vi "Prepare Data for LSL.vi"(10 "Data Cluster":T1={"Status"="", "LSL Streaming"=FALSE, "channel_format"=1, "outlet"=0, "streaminfo"=0, "xml_ptr"=0, "LSL Listeners"=0, "LSL Listeners Query Counter"=0, "Data Chunk "={"counter"=0, "Data"=[]}, "Ch En Map"=[]} {"channel_format" items=["cft_float32"=1, "cft_double64"=2, "cft_string"=3, "cft_int32"=4, "cft_int16"=5, "cft_int8"=6, "cft_int64"=7, "cft_undefined"=0]}, 11 "WiBCI16T Data":T6 {"Reg Map"."ADS2" format="%x"; "Reg Map"."ADS1" format="%x"}) -> (2 "Data Chunk Size":i32, 3 "Prepared Data Array":dbl[][](array[numeric]))   [LabVIEW 2016, in "Lab Streaming Layer.lvlib"]
uses:
  Lab Streaming Layer.lvlib
  Acquisition/WiBCI16T_Data.ctl
  Acquisition/WiBCI16T_Status.ctl
  Acquisition/Reg_Map.ctl
  Module Data--cluster.ctl
  Custom Controls/lsl_channel_format.ctl
  Custom Controls/lsl_outlet.ctl
  Custom Controls/lsl_streaminfo.ctl
  Custom Controls/lsl_xml_ptr.ctl
  Acquisition/Acquisition.lvlib
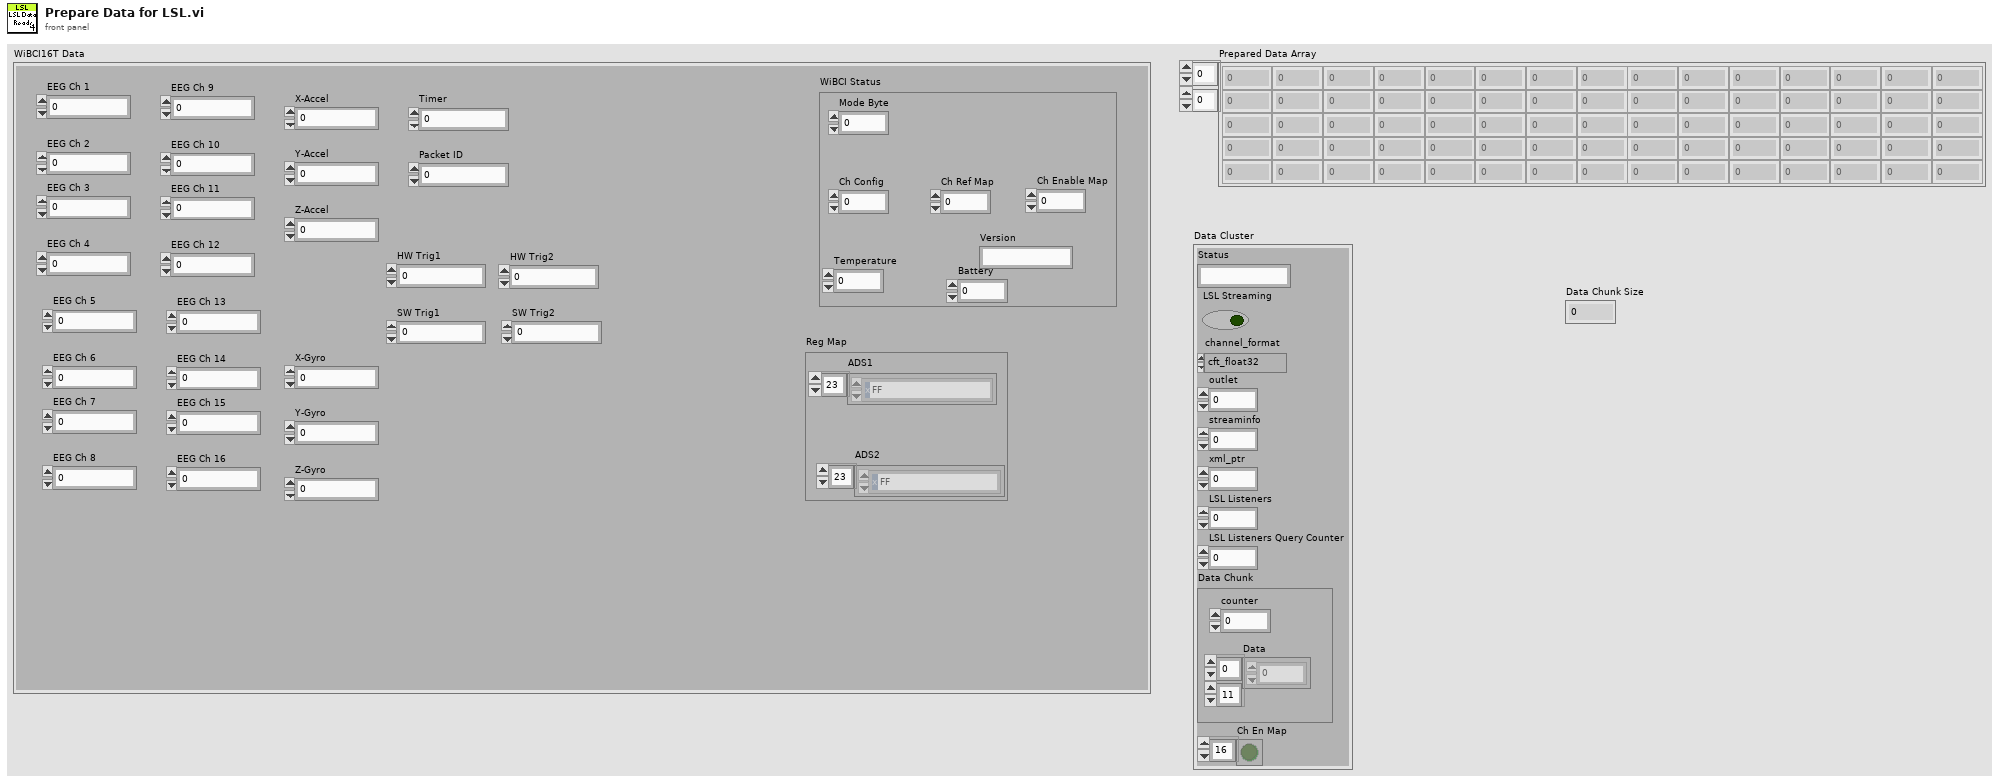
[diagram p1: front panel]
types:
  T1 = typedef "Lab Streaming Layer.lvlib/Module Data--cluster.ctl" = cluster{"Status":string, "LSL Streaming":bool, "channel_format":T2, "outlet":T3, "streaminfo":T4, "xml_ptr":T5, "LSL Listeners":i32, "LSL Listeners Query Counter":i32, "Data Chunk ":cluster{"counter":u8, "Data":dbl[][]}, "Ch En Map":bool[]}
  T2 = typedef "Lab Streaming Layer.lvlib/lsl_channel_format.ctl" = u32
  T3 = typedef "Lab Streaming Layer.lvlib/lsl_outlet.ctl" = u64
  T4 = typedef "Lab Streaming Layer.lvlib/lsl_streaminfo.ctl" = u64
  T5 = typedef "Lab Streaming Layer.lvlib/lsl_xml_ptr.ctl" = u64
  T6 = typedef "Acquisition.lvlib/WiBCI16T_Data.ctl" = cluster{"EEG Ch 1":dbl, "EEG Ch 2":dbl, "EEG Ch 3":dbl, "EEG Ch 4":dbl, "EEG Ch 5":dbl, "EEG Ch 6":dbl, "EEG Ch 7":dbl, "EEG Ch 8":dbl, "EEG Ch 9":dbl, "EEG Ch 10":dbl, "EEG Ch 11":dbl, "EEG Ch 12":dbl, "EEG Ch 13":dbl, "EEG Ch 14":dbl, "EEG Ch 15":dbl, "EEG Ch 16":dbl, "X-Accel":i16, "Y-Accel":i16, "Z-Accel":i16, "X-Gyro":i16, "Y-Gyro":i16, "Z-Gyro":i16, "Timer":u32, "Packet ID":u32, "HW Trig1":u8, "SW Trig1":i8, "HW Trig2":u8, "SW Trig2":i8, "WiBCI Status":T7, "Reg Map":T8}
  T7 = typedef "Acquisition.lvlib/WiBCI16T_Status.ctl" = cluster{"Mode Byte":u8, "Ch Config":u8, "Ch Ref Map":u16, "Ch Enable Map":u16, "Temperature":sgl, "Battery":u8, "Version":string}
  T8 = typedef "Acquisition.lvlib/Reg_Map.ctl" = cluster{"ADS1":u8[], "ADS2":u8[]}
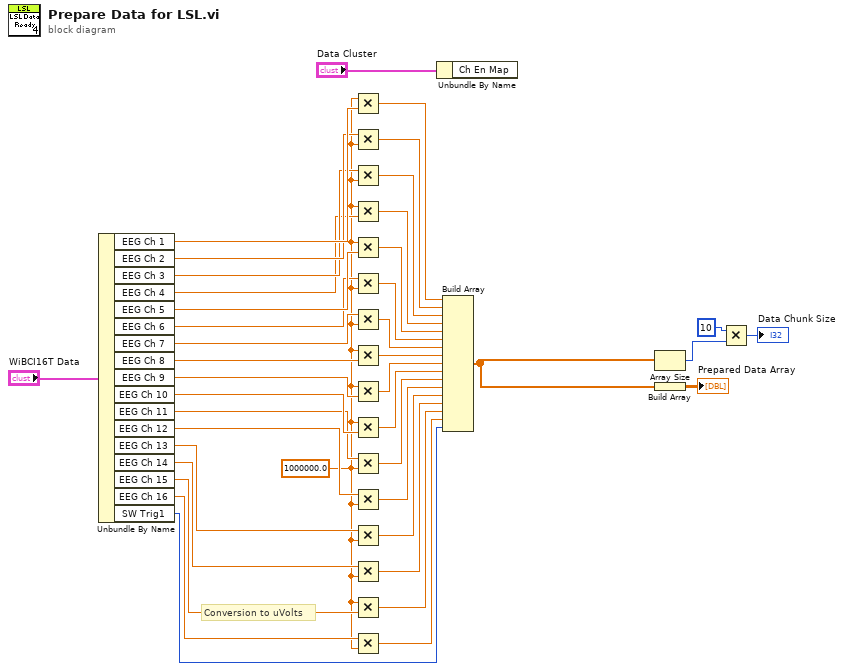
[diagram p0: block diagram]
diagram:
  w5 = 1000000.0 ("x")
  # "Conversion to uVolts"
  n1 = Unbundle By Name("WiBCI16T Data") -> ("EEG Ch 1"=w25:dbl, "EEG Ch 2"=w24:dbl, "EEG Ch 3"=w23:dbl, "EEG Ch 4"=w22:dbl, "EEG Ch 5"=w21:dbl, "EEG Ch 6"=w20:dbl, "EEG Ch 7"=w19:dbl, "EEG Ch 8"=w18:dbl, "EEG Ch 9"=w17:dbl, "EEG Ch 10"=w16:dbl, "EEG Ch 11"=w15:dbl, "EEG Ch 12"=w14:dbl, "EEG Ch 13"=w13:dbl, "EEG Ch 14"=w12:dbl, "EEG Ch 15"=w11:dbl, "EEG Ch 16"=w10:dbl, "SW Trig1"=w1:i8)
  n2 = Multiply(x=w5, y=w25) -> (x*y=w9:dbl)
  n3 = Multiply(x=w24, y=w5) -> (x*y=w8:dbl)
  n4 = Multiply(x=w23, y=w5) -> (x*y=w26:dbl)
  n5 = Multiply(x=w5, y=w22) -> (x*y=w27:dbl)
  n6 = Multiply(x=w5, y=w21) -> (x*y=w28:dbl)
  n7 = Multiply(x=w20, y=w5) -> (x*y=w29:dbl)
  n8 = Multiply(x=w19, y=w5) -> (x*y=w30:dbl)
  n9 = Multiply(x=w5, y=w18) -> (x*y=w31:dbl)
  n10 = Multiply(x=w5, y=w17) -> (x*y=w32:dbl)
  n11 = Multiply(x=w5, y=w16) -> (x*y=w33:dbl)
  n12 = Multiply(x=w15, y=w5) -> (x*y=w34:dbl)
  n13 = Multiply(x=w14, y=w5) -> (x*y=w35:dbl)
  n14 = Multiply(x=w13, y=w5) -> (x*y=w36:dbl)
  n15 = Multiply(x=w12, y=w5) -> (x*y=w38:dbl)
  n16 = Multiply(x=w5, y=w11) -> (x*y=w37:dbl)
  n17 = Multiply(x=w10, y=w5) -> (x*y=w39:dbl)
  n18 = Unbundle By Name("Data Cluster") -> ()  [unwired: 1 out]
  n19 = Build Array(w9, w8, w26, w27, w28, w29, w30, w31, w32, w33, w34, w35, w36, w38, w37, w39, w1) -> (w6:dbl[])
  n20 = Array Size(array=w6) -> (size(s)=w4:i32)
  n21 = Build Array(w6) -> (→"Prepared Data Array":dbl[][])
  n22 = Multiply(x=10, y=w4) -> (x*y=→"Data Chunk Size":i32)
